vi "Check Start Point and Length.vi"(8 "error in (no error)":errorcluster, 9 "Total Samples in TDMS (10000)":i32=10000, 10 "Start Point (0)":i32, 11 "Length (1000)":i32=1000) -> (0 "error out":errorcluster, 3 "Actual Points":i32)   [LabVIEW 2013, in "Agilent 90000 Series.lvlib"]
doc: "Returns the actual points by the number of samples, offset and total points in the instrument memory buffer."
uses:
  Agilent 90000 Series.lvlib
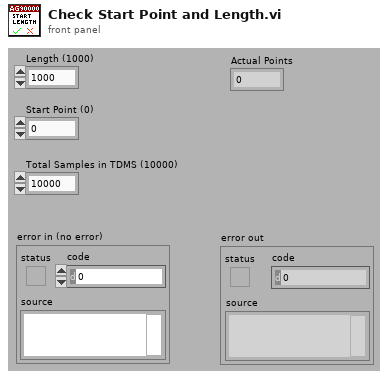
[diagram p1: front panel]
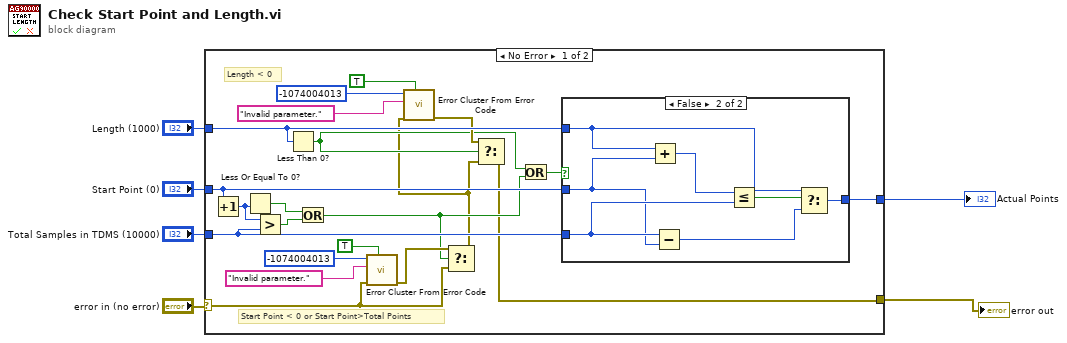
[diagram p0: block diagram]
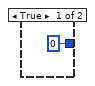
[diagram p2: hidden frame]
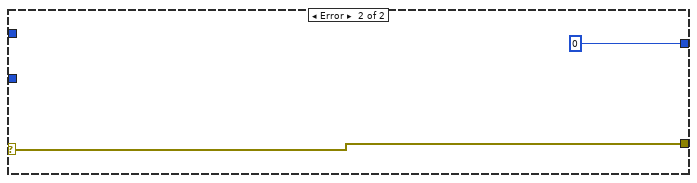
[diagram p3: hidden frame]
diagram:
  n1 = case shown="No Error" "error in (no error)" {
    selector: "error in (no error)" -> [w8 w37]
    tunnel: "Total Samples in TDMS (10000)" -> [w25 _]
    tunnel: "Start Point (0)" -> [w26 _]
    tunnel: "Length (1000)" -> [w18 _]
    tunnel: [w27 0 ("Number of Samples")] -> w3
    tunnel: [w10 w37] -> w1
    frame No Error {
      # "Start Point < 0 or Start Point>Total Points"
      # "Length < 0"
      n2 = Increment(x=w26) -> (x+1=w9:i32)
      n3 = Less Or Equal To 0?(x=w9) -> (x <= 0?=w24:bool)
      n4 = Greater?(x=w9, y=w25) -> (0:w23:bool)
      n5 = Less Than 0?(x=w18) -> (x < 0?=w13:bool)
      n6 = Or(x=w24, y=w23) -> (x .or. y?=w12:bool)
      n7 = call <vilib>:"Error Cluster From Error Code.vi"("show call chain? (False)"=TRUE, "error in (no error)"=w8, "error message (\"\")"="Invalid parameter." ("error message (\"\")"), "error code (0)"=-1074004013) -> ("error out"=w19:errorcluster)  [unwired: 5 in]
      n8 = Select(t=w19, s=w12, f=w8) -> (s? t:f=w7:errorcluster)
      n9 = call <vilib>:"Error Cluster From Error Code.vi"("show call chain? (False)"=TRUE, "error in (no error)"=w7, "error message (\"\")"="Invalid parameter." ("error message (\"\")"), "error code (0)"=-1074004013) -> ("error out"=w14:errorcluster)  [unwired: 5 in]
      n10 = Select(t=w14, s=w13, f=w7) -> (s? t:f=w10:errorcluster)
      n11 = Or(x=w13, y=w12) -> (x .or. y?=w11:bool)
      n12 = case shown="False" w11 {
        tunnel: [0 ("Number of Samples") w35] -> w27
        tunnel: w26 -> [_ w29]
        tunnel: w25 -> [_ w32]
        tunnel: w18 -> [_ w31]
        frame True {
        }
        frame False {
          n13 = Add(x=w31, y=w29) -> (x+y=w30:i32)
          n14 = Subtract(x=w32, y=w29) -> (x-y=w33:i32)
          n15 = Less Or Equal?(x=w30, y=w32) -> (x <= y?=w34:bool)
          n16 = Select(t=w31, s=w34, f=w33) -> (s? t:f=w35:i32)
        }
      }
    }
    frame Error {
    }
  }
  "Actual Points" <- w3
  "error out" <- w1
